vi "Board Alarm Status.vi"(8 "error in (no error)":errorcluster, 11 "BoardHandle":T2) -> (0 "error out":errorcluster, 1 "Board status (decimal value)":i32, 2 "Board status":T1, 3 "BoardHandle out":T2)   [LabVIEW 2009, in "CAEN PSM.lvlib"]
doc: "This function reports board alarm status."
uses:
  <instrlib>/CAEN PSM/CAEN PSM.lvlib
  <instrlib>/CAEN PSM/Private/BoardHandle.ctl
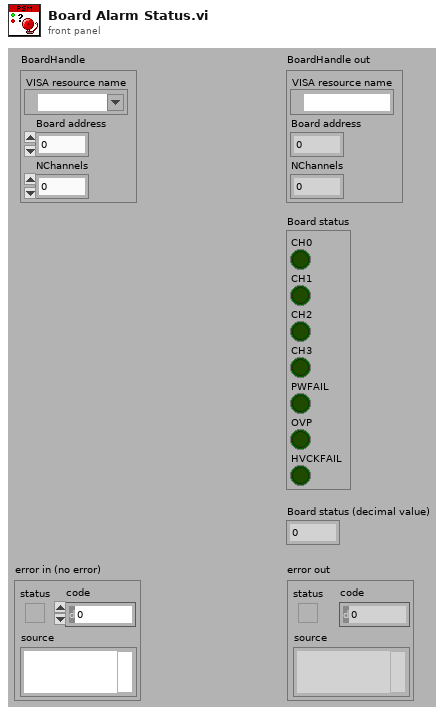
[diagram p1: front panel]
types:
  T1 = cluster{"CH0":bool, "CH1":bool, "CH2":bool, "CH3":bool, "PWFAIL":bool, "OVP":bool, "HVCKFAIL":bool}
  T2 = typedef "CAEN PSM.lvlib/BoardHandle.ctl" = cluster{"VISA resource name":refnum<visa-resource-name>, "Board address":u8, "NChannels":u8}
  T3 = cluster{"Boolean array[0]":bool, "Boolean array[1]":bool, "Boolean array[2]":bool, "Boolean array[3]":bool, "Boolean array[4]":bool, "Boolean array[5]":bool, "Boolean array[6]":bool}
  T4 = cluster{"Boolean array":cluster{"Boolean array[0]":bool, "Boolean array[1]":bool, "Boolean array[2]":bool, "Boolean array[3]":bool, "Boolean array[4]":bool, "Boolean array[5]":bool, "Boolean array[6]":bool}}[]
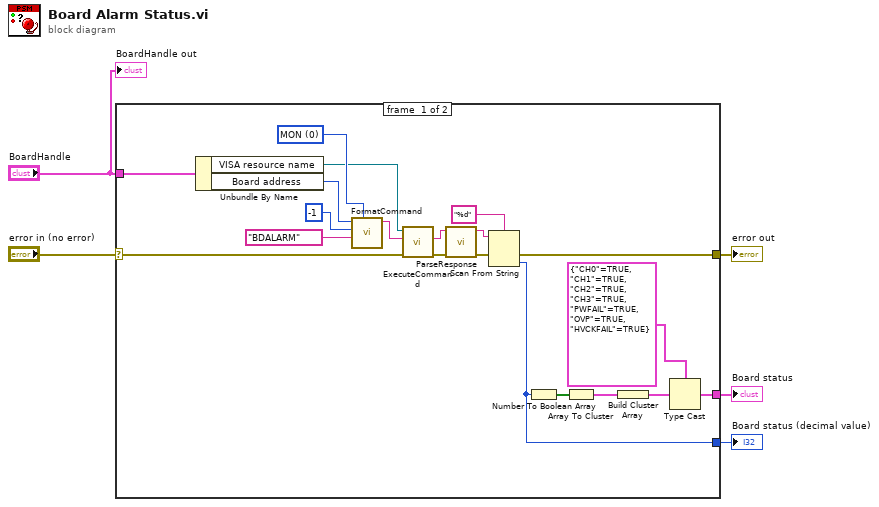
[diagram p0: block diagram]
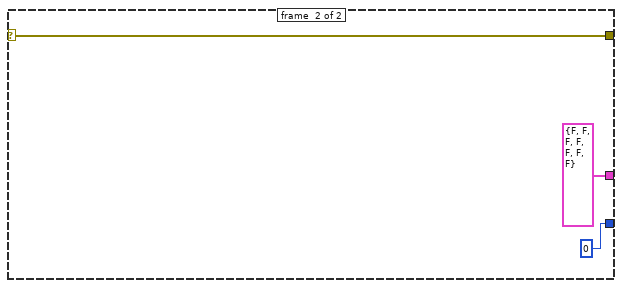
[diagram p2: hidden frame]
diagram:
  n1 = case shown="No Error" "error in (no error)" {
    selector: "error in (no error)" -> [w18 w28]
    tunnel: [w13 w28] -> w4
    tunnel: "BoardHandle" -> [w19 _]
    tunnel: [w7 T1 {"CH0"=FALSE, "CH1"=FALSE, "CH2"=FALSE, "CH3"=FALSE, "PWFAIL"=FALSE, "OVP"=FALSE, "HVCKFAIL"=FALSE} ("input cluster")] -> w2
    tunnel: [w6 0] -> w1
    frame #0 {
      w24 = u8 0 items=["MON", "SET"] ("CMD")
      n2 = Unbundle By Name(w19) -> ("VISA resource name"=w23:refnum<visa-resource-name>, "Board address"=w25:u8)
      n3 = call <instrlib>:"FormatCommand.vi"("CMD (MON)"=w24, "PAR"="BDALARM", "CH"=i8 -1, "BD (0)"=w25) -> ("cmd"=w22:string)  [unwired: 7 in]
      n4 = call <instrlib>:"ExecuteCommand.vi"("error in (no error)"=w18, "Command"=w22, "VISA resource name"=w23) -> ("error out"=w21:errorcluster, "Response"=w20:string)  [unwired: 6 in, 1 out]
      n5 = call <instrlib>:"ParseResponse.vi"("error in (no error)"=w21, "Response"=w20) -> ("error out"=w15:errorcluster, "val"=w16:string)  [unwired: 6 in, 2 out]
      n6 = Scan From String(format string="%d", input string=w16, error in=w15) -> (error out=w13:errorcluster, output 1=w6:i32)  [unwired: 2 in, 2 out]
      n7 = Number To Boolean Array(number=w6) -> (Boolean array=w10:bool[])
      n8 = Array To Cluster(array=w10) -> (cluster=w9:T3)
      n9 = Build Cluster Array(w9) -> (w14:T4)
      n10 = Type Cast(type=T1 {"CH0"=TRUE, "CH1"=TRUE, "CH2"=TRUE, "CH3"=TRUE, "PWFAIL"=TRUE, "OVP"=TRUE, "HVCKFAIL"=TRUE} ("input cluster"), x=w14) -> (*(type *) &x=w7:T1)
    }
    frame #1 {
    }
  }
  "error out" <- w4
  "Board status" <- w2
  "Board status (decimal value)" <- w1
  "BoardHandle out" <- "BoardHandle"
